vi "ratio_pixel2mil.vi"(10 "max corner in":dbl[][](array[numeric]), 11 "side perimeter (mm)":dbl) -> (3 "ratio":dbl)   [LabVIEW 2017]
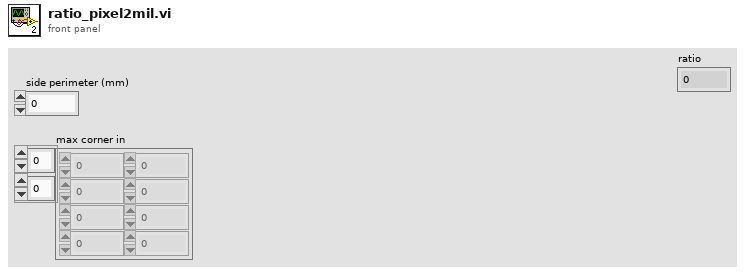
[diagram p1: front panel]
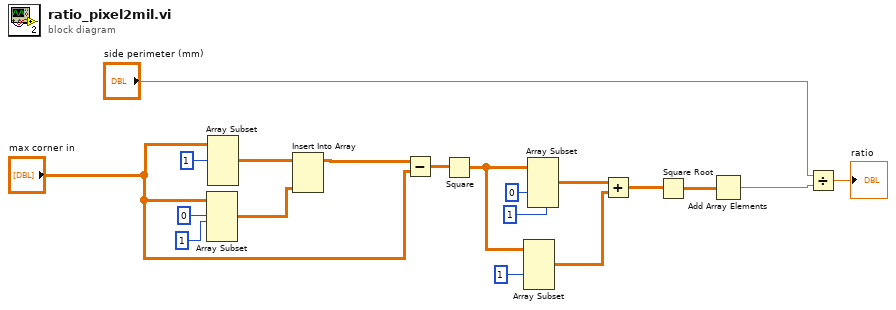
[diagram p0: block diagram]
diagram:
  n1 = Array Subset(array="max corner in", index (row)=0 ("length"), length (row)=1 ("length")) -> (w15:dbl[][])  [unwired: 2 in]
  n2 = Array Subset(array="max corner in", index (row)=1 ("index")) -> (w16:dbl[][])  [unwired: 3 in]
  n3 = Insert Into Array "Insert Into Array"(array=w16, new element=w15) -> (w14:dbl[][])  [unwired: 2 in]
  n4 = Subtract(x=w14, y="max corner in") -> (x-y=w12:dbl[][])
  n5 = Square(x=w12) -> (x^2=w8:dbl[][])
  n6 = Array Subset(array=w8, index (col)=1 ("index")) -> (w6:dbl[][])  [unwired: 3 in]
  n7 = Array Subset(array=w8, index (col)=0 ("index"), length (col)=1 ("index")) -> (w7:dbl[][])  [unwired: 2 in]
  n8 = Add(x=w7, y=w6) -> (x+y=w5:dbl[][])
  n9 = Square Root(x=w5) -> (sqrt(x)=w4:dbl[][])
  n10 = Add Array Elements(numeric array=w4) -> (sum=w1:dbl)
  n11 = Divide(x="side perimeter (mm)", y=w1) -> (x/y=→"ratio":dbl)
